vi "Main.vi"() -> ()   [LabVIEW 2019]
doc: "The myRIO Project template acquires acceleration data from the onboard accelerometer and displays the changes of acceleration values in a waveform chart."
uses:
  <vilib>/Platform/TimedLoop/XDataNode/timing_clust.ctl
  <vilib>/Platform/TimedLoop/XDataNode/nitl_modes.ctl
  <vilib>/Platform/TimedLoop/XDataNode/wakeup.ctl
  <vilib>/myRIO/Common/Instrument Driver Framework/myRIO v1.0/UART/vis/myRIO v1.0 Close UART.vi
  <vilib>/myRIO/Common/Instrument Driver Framework/Utilities/vis/FPGA Ref Manager.vi
  <vilib>/myRIO/Common/Instrument Driver Framework/myRIO v1.0/myRIO v1.0 Reset FPGA.vi
  <vilib>/myRIO/Common/Instrument Driver Framework/myRIO v1.0/IRQ/vis/myRIO v1.0 IRQ Info FGV.vi
  <vilib>/myRIO/Common/Instrument Driver Framework/myRIO v1.0/IRQ/vis/myRIO v1.0 Timer IRQ Info FGV.vi
  <vilib>/myRIO/Common/Instrument Driver Framework/myRIO v1.0/IRQ/vis/myRIO v1.0 ISR Agent.vi
  <vilib>/myRIO/Instrument Drivers/Utilities/vis/Reset Index.vi
  <vilib>/myRIO/Common/Instrument Driver Framework/myRIO v1.0/Resource Manager/vis/myRIO v1.0 Block Write Resource Manager.vi
  <vilib>/platform/TimedLoop/XDataNode/XDataNode.xnode
  <vilib>/myRIO/Instrument Drivers/Utilities/Utilities.lvlib
  <vilib>/Platform/TimedLoop/XDataNode/XDNodeRunTimeDep.lvlib
panel:
  out "Motor Controls":dbl[](array[numeric])
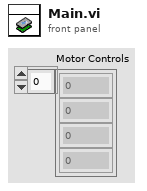
[diagram p1: front panel]
types:
  T1 = cluster{"proportional gain (Kc)":dbl, "integral time (Ti, min)":dbl, "derivative time (Td, min)":dbl}[]
  T2 = typedef "XDNodeRunTimeDep.lvlib/timing_clust.ctl" = cluster{"Expected End [f-1]":u64, "Actual End [f-1]":u64, "Finished Late? [f-1]":bool, "Expected End [i-1]":u64, "Actual End [i-1]":u64, "Finished Late? [i-1]":bool, "Expected Start [i]":u64, "Actual Start [i]":u64, "Expected Start [f]":u64, "Actual Start [f]":u64, "Source Name":string, "Structure Name":string, "Period":i64, "Deadline":i64, "Offset":i64, "Start":i64, "Priority":i32, "Timeout":i32, "Mode":T3, "Wakeup Reason":T4, "Error":errorcluster, "Source Type":string, "Secondary Source Type":string, "Global End Time":u64, "Global Start Time":u64, "Frame Duration":u64, "Iteration Duration":u64, "Assigned CPU":i32, "I/O Scan Engine Mode":u32}
  T3 = typedef "XDNodeRunTimeDep.lvlib/nitl_modes.ctl" = enum32{"No Change", "Process missed periods, maintain original phase", "Discard missed periods, maintain original phase", "Process missed periods, ignore original phase", "Discard missed periods, ignore original phase"}
  T4 = typedef "XDNodeRunTimeDep.lvlib/wakeup.ctl" = enum32{"Normal", "Aborted", "Asynchronous wakeup", "Timing source error", "Timed loop error", "Timeout"}
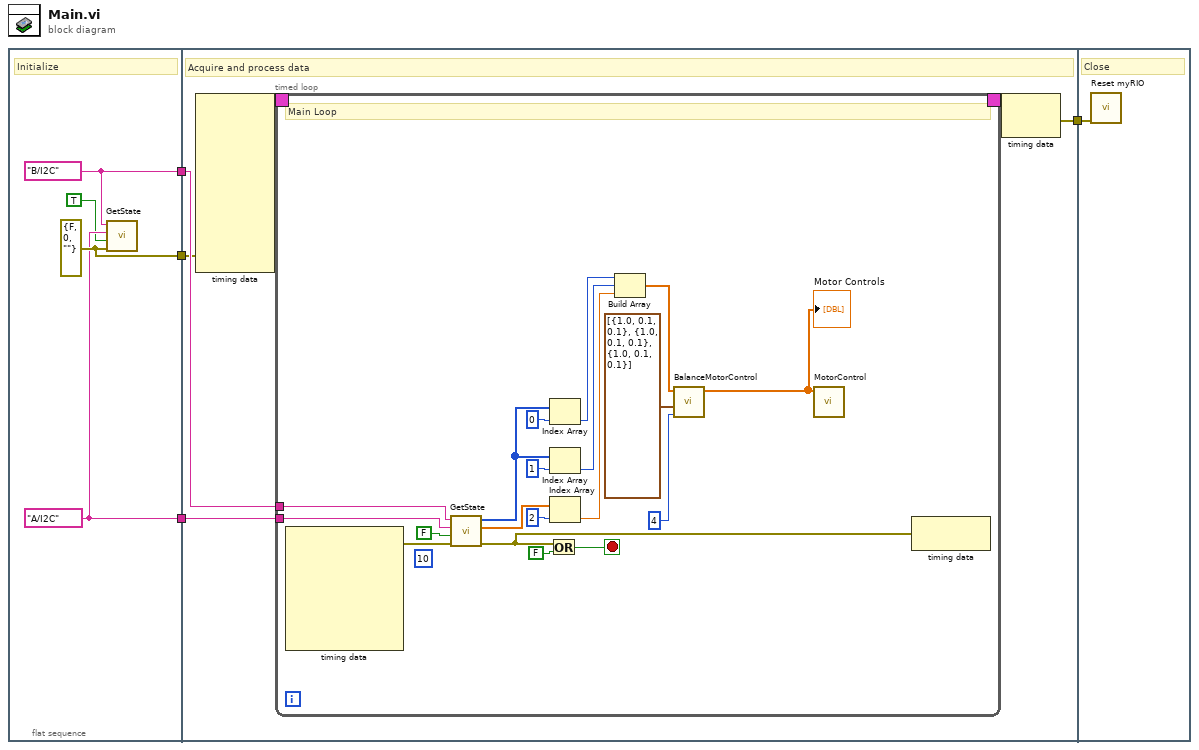
[diagram p0: block diagram]
diagram:
  n1 = flat-sequence {
    tunnel: [w8] -> w4
    tunnel: [w6] -> w2
    tunnel: [w7] -> w1
    tunnel: w4 -> [w10]
    tunnel: [w9] -> w3
    tunnel: w2 -> [w14]
    tunnel: w1 -> [w13]
    tunnel: w3 -> [w44]
    frame #0 {
      w7 = tag "A/I2C" ("IMU Channel")
      w6 = tag "B/I2C" ("LIDAR Channel")
      w8 = errorcluster {"status"=FALSE, "code"=0, "source"=""} ("error in (no error)")
      # "Initialize"
      n2 = call "GetState.vi"("error in (no error)"=w8, "Calibrate?"=TRUE, "IMU Channel"=w7, "LIDAR Channel"=w6) -> ()  [unwired: 2 in, 4 out]
    }
    frame #1 {
      # "Acquire and process data"
      n3 = node-c288(w10) -> (w12:T2)  [unwired: 9 in]
      n4 = timed-loop {
        tunnel: w14 -> [w31]
        tunnel: w13 -> [w30]
        timing: w12 -> [_]
        timing-out: [_] -> w11
        stop <- w33 stop-if-true
        (unwired) u32 10 ("milliseconds to wait")
        # "Main Loop"
        n5 = node-c288() -> (w15:errorcluster)  [unwired: 1 in, 6 out]
        n6 = call "GetState.vi"("error in (no error)"=w15, "Calibrate?"=FALSE, "IMU Channel"=w30, "LIDAR Channel"=w31) -> ("error out"=w16:errorcluster, "Angular Velocity"=w27:dbl[], "imu accel"=w25:i16[])  [unwired: 2 in, 1 out]
        n7 = Or(x=w16, y=FALSE) -> (x .or. y?=w33:bool)
        n8 = Index Array(array=w25, index=0) -> (element=w20:i16)
        n9 = Index Array(array=w25, index=1) -> (element=w19:i16)
        n10 = Index Array(array=w27, index=2) -> (element=w18:dbl)
        n11 = Build Array(w20, w19, w18) -> (w22:dbl[])
        n12 = call "BalanceMotorControl.vi"("Number of Motors"=i16 4, "PID Gains"=T1 [{"proportional gain (Kc)"=1.0, "integral time (Ti, min)"=0.1, "derivative time (Td, min)"=0.1}, {"proportional gain (Kc)"=1.0, "integral time (Ti, min)"=0.1, "derivative time (Td, min)"=0.1}, {"proportional gain (Kc)"=1.0, "integral time (Ti, min)"=0.1, "derivative time (Td, min)"=0.1}], "Gx, Gy, wz"=w22) -> ("Motor Controls"=w17:dbl[])  [unwired: 8 in]
        "Motor Controls" <- w17
        n13 = call "MotorControl.vi"("Array"=w17) -> ()  [unwired: 11 in]
        n14 = node-c288(w16) -> ()  [unwired: 1 out]
      }
      n15 = node-c288(w11) -> (w9:errorcluster)
    }
    frame #2 {
      # "Close"
      n16 = call <vilib>:"Reset myRIO.vi"("error in (no error)"=w44) -> ()  [unwired: 10 in, 1 out]
    }
  }
